vi "MC5e Add Squad to Unit.vi"(8 "error in":errorcluster, 9 "# to add":u16, 10 "Squad Index":i32, 11 "Unit Index":i32) -> (0 "error out":errorcluster)   [LabVIEW 2020]
uses:
  MC5e Squad_Manager_Modes.ctl
  MC5e Unit_Manager_Modes.ctl
  MC5e Editor modes.ctl
panel:
  out "squad index":i32
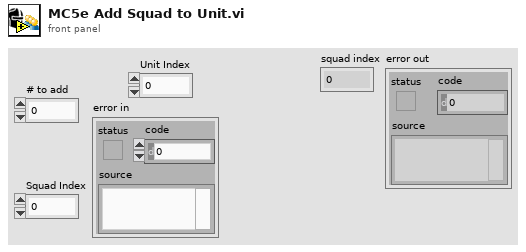
[diagram p1: front panel]
types:
  T1 = typedef "MC5e Editor modes.ctl" = enum16{"Add New", "Copy Selected", "Delete Selected", "Edit Selected"}
  T2 = typedef "MC5e Unit_Manager_Modes.ctl" = enum16{"Initialize", "Add Unit", "Delete Unit", "Get Unit", "Load Set", "Replace Unit"}
  T3 = typedef "MC5e Squad_Manager_Modes.ctl" = enum16{"Initialize", "Add Squad", "Delete Squad", "Get Squad", "Replace Squad", "Load Set"}
  T4 = typedef "MC5e Squad_Info.ctl" = cluster{"Squad Name":string, "# Soldiers":u16, "Battle Rating":u16, "Flying":bool, "Mounted":bool, "Speed":u16, "Range":u16, "Morale":i32, "Max Endurance":u16, "Current Endurance":i32, "Size":T5, "Space Taken":u16, "Difficult Terrain":i32[], "CR":u16, "Special / Notes":string}
  T5 = typedef "MC5e Size_Categories.ctl" = enum16{"Tiny", "Small", "Medium", "Large", "Huge", "Gargantuan"}
  T6 = typedef "MC5e Unit.ctl" = cluster{"Unit Fatigue Level":enum16{"Not Fatigued", "Fatigued", "Seriously Fatigued"}, "Flying Unit":bool, "Mounted Unit":bool, "Defending from Stronghold":bool, "Difficult Terrain Types":T7, "Squads in Unit":T4[], "Unit Info":T8, "Range":i32, "BR":i32, "Speed":i32, "Morale":i32, "Current BR":i32, "Location":T9, "Capacity %":i32}
  T7 = typedef "MC5e Terrain types.ctl" = i32[]
  T8 = typedef "MC5e Unit Header.ctl" = cluster{"Unit Name":string, "Unit Commander":string, "Morale Mod":i32, "BR Mod":i32, "Defense Mod":i32, "Speed Mod":i32, "Unit Notes":string, "Attack Mod":i32, "Unit Wins+ Losses-":i32, "Commander Charisma Bonus":i32}
  T9 = typedef "Location.ctl" = cluster{"X coordinate":dbl, "Y coordinate":dbl}
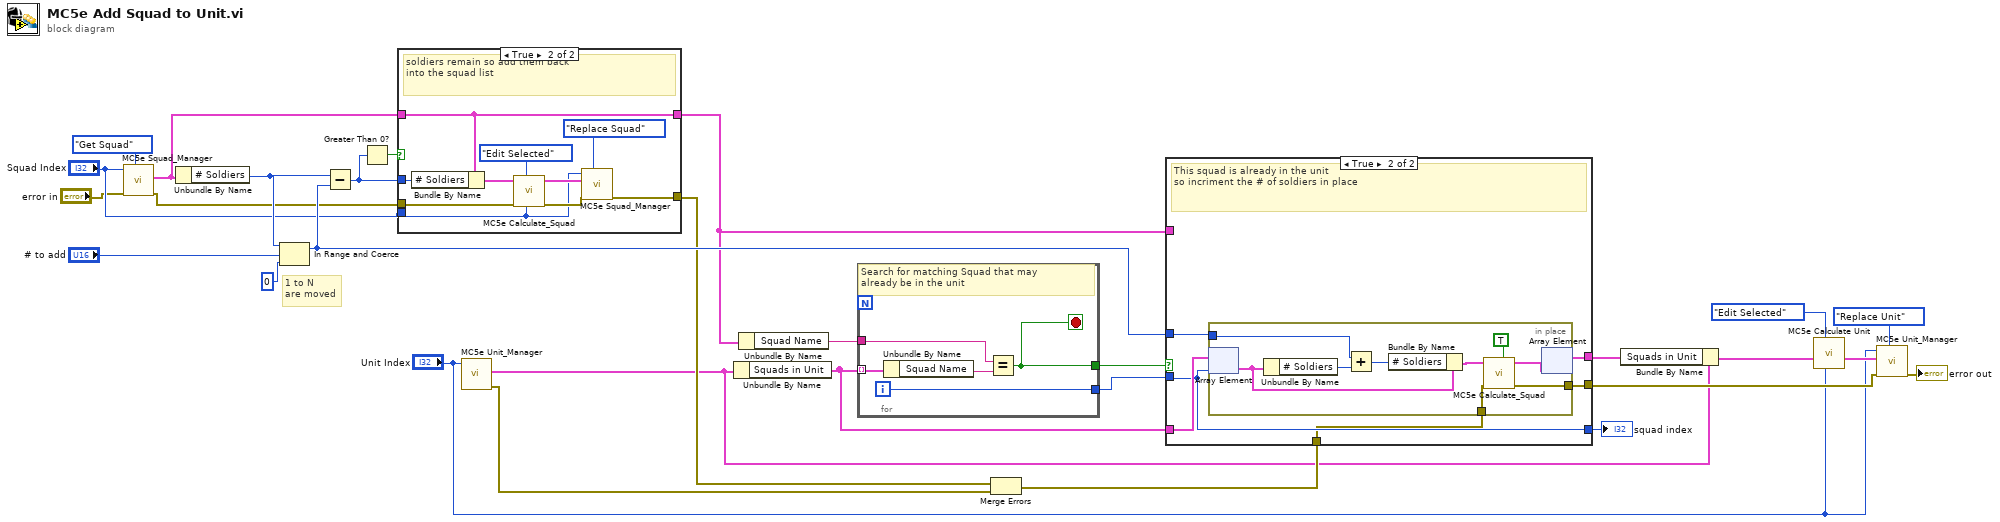
[diagram p0: block diagram]
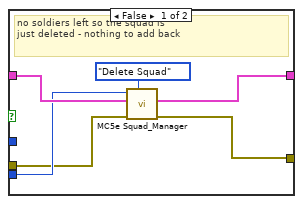
[diagram p2: hidden frame]
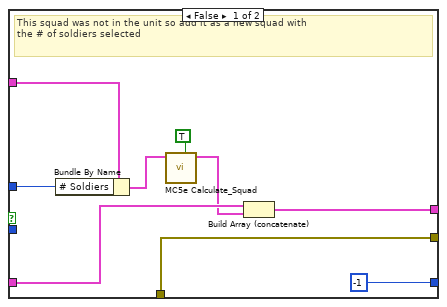
[diagram p3: hidden frame]
diagram:
  # "1 to N\nare moved"
  n1 = call "MC5e Squad_Manager.vi"("Mode (Get)"=MC5e_Squad_Manager_Modes."Get Squad", "error in"="error in", "index (get/delete/replace)"="Squad Index") -> ("error out"=w7:errorcluster, "Squad"=w18:T4)  [unwired: 5 in, 2 out]
  n2 = Unbundle By Name(w18) -> ("# Soldiers"=w28:u16)
  n3 = In Range and Coerce(upper limit=w28, x="# to add", lower limit=u16 0) -> (coerced(x)=w21:u16)  [unwired: 1 out]
  n4 = Subtract(x=w28, y=w21) -> (x-y=w17:u16)
  n5 = Greater Than 0?(x=w17) -> (x > 0?=w16:bool)
  n6 = case shown="True" w16 {
    tunnel: w17 -> [_ w44]
    tunnel: w18 -> [w35 w43]
    tunnel: [w31 w43] -> w2
    tunnel: "Squad Index" -> [w34 w36]
    tunnel: [w32 w39] -> w10
    tunnel: w7 -> [w33 w37]
    frame False {
      # "no soldiers left so the squad is\njust deleted - nothing to add back"
      n7 = call "MC5e Squad_Manager.vi"("Mode (Get)"=MC5e_Squad_Manager_Modes."Delete Squad", "error in"=w33, "Squad in (add/replace)"=w35, "index (get/delete/replace)"=w34) -> ("error out"=w32:errorcluster, "Squad"=w31:T4)  [unwired: 4 in, 2 out]
    }
    frame True {
      # "soldiers remain so add them back\ninto the squad list"
      n8 = Bundle By Name(cluster=w43, "# Soldiers"=w44) -> (w42:T4)
      n9 = call "MC5e Calculate_Squad.vi"("index"=w36, "Mode"=MC5e_Editor_modes."Edit Selected", "error in"=w37, "Input Squad"=w42) -> ("error out"=w38:errorcluster, "output squad"=w41:T4)  [unwired: 5 in, 1 out]
      n10 = call "MC5e Squad_Manager.vi"("Mode (Get)"=MC5e_Squad_Manager_Modes."Replace Squad", "error in"=w38, "Squad in (add/replace)"=w41, "index (get/delete/replace)"=w36) -> ("error out"=w39:errorcluster)  [unwired: 4 in, 3 out]
    }
  }
  n11 = call "MC5e Unit_Manager.vi"("index (get/delete/replace)"="Unit Index") -> ("error out"=w8:errorcluster, "Unit"=w3:T6)  [unwired: 7 in, 2 out]
  n12 = Unbundle By Name(w3) -> ("Squads in Unit"=w24:T4[])
  n13 = Unbundle By Name(w2) -> ("Squad Name"=w25:string)
  n14 = for {
    tunnel: w24 -> [w50] mode=indexing
    tunnel: w25 -> [w48]
    tunnel: [w47] -> w23
    tunnel: [w46] -> w22
    i -> [w46]
    stop <- w47 stop-if-true
    # "Search for matching Squad that may\nalready be in the unit"
    n15 = Unbundle By Name(w50) -> ("Squad Name"=w49:string)
    n16 = Equal?(x=w48, y=w49) -> (x = y?=w47:bool)
  }
  n17 = Merge Errors(w10, w8) -> (w9:errorcluster)
  n18 = case shown="True" w23 {
    tunnel: w24 -> [w57 w65]
    tunnel: w22 -> [_ w63]
    tunnel: w21 -> [w58 w64]
    tunnel: [w56 w60] -> w1
    tunnel: [-1 w63] -> w19
    tunnel: [w55 w62] -> w11
    tunnel: w9 -> [w55 w61]
    tunnel: w2 -> [w54 _]
    frame False {
      # "This squad was not in the unit so add it as a new squad with\nthe # of soldiers selected"
      n19 = Bundle By Name(cluster=w54, "# Soldiers"=w58) -> (w53:T4)
      n20 = call "MC5e Calculate_Squad.vi"("Skip Name Check (F)"=TRUE, "Input Squad"=w53) -> ("output squad"=w52:T4)  [unwired: 7 in, 2 out]
      n21 = Build Array (concatenate)(w57, w52) -> (w56:T4[])
    }
    frame True {
      # "This squad is already in the unit\nso incriment the # of soldiers in place"
      n22 = in-place {
        in-place-border: w64 -> [w73]
        in-place-border: [w68] -> w62
        in-place-border: w61 -> [w67]
        n23 = in-place-array #1(w65, w63) -> (w72:T4)
        n24 = Unbundle By Name(w72) -> ("# Soldiers"=w74:u16)
        n25 = Add(x=w73, y=w74) -> (x+y=w71:u16)
        n26 = Bundle By Name(cluster=w72, "# Soldiers"=w71) -> (w70:T4)
        n27 = call "MC5e Calculate_Squad.vi"("Skip Name Check (F)"=TRUE, "error in"=w67, "Input Squad"=w70) -> ("error out"=w68:errorcluster, "output squad"=w69:T4)  [unwired: 6 in, 1 out]
        n28 = in-place-array #1(w69) -> (w60:T4[])  [unwired: 1 out]
      }
    }
  }
  "squad index" <- w19
  n29 = Bundle By Name(cluster=w3, "Squads in Unit"=w1) -> (w15:T6)
  n30 = call "MC5e Calculate Unit.vi"("index"="Unit Index", "Mode"=MC5e_Editor_modes."Edit Selected", "Unit In"=w15) -> ("Unit Out"=w14:T6)  [unwired: 5 in, 3 out]
  n31 = call "MC5e Unit_Manager.vi"("Mode (Get)"=MC5e_Unit_Manager_Modes."Replace Unit", "error in"=w11, "Unit In (Add/Replace)"=w14, "index (get/delete/replace)"="Unit Index") -> ("error out"=→"error out":errorcluster)  [unwired: 4 in, 3 out]
